vi "Check Overflows.vi"(0 "ignore overflow?":bool, 1 "clear overflow?":bool, 2 "reset":bool, 5 "overflow":bool, 7 "samples per cycle (SPC)":u32, 9 "input valid":bool, 11 "group delay (samples)":fxp<+,64,32> format="%#_42g") -> (4 "overflow?":bool)   [LabVIEW 2023]
doc: "<b>Pipeline Delay = 0</b>\n\nthis VI checks for overflows based on the input configuration. the 'overflow' is latched and must be cleared via 'clear overflow?' or 'reset'.\n\n<b>clear overflow?:</b> clear the overflow status. will immediately affect the output 'overflow?'.\n\n<b>ignore overflows:</b> indicates that overflows detected in the current cycle should be suppressed.\n\n<b>group delay (samples):</b> used to define the number of samples to ignore for unwanted DSP transients. if set to constant 0, group delay logic will not be placed."
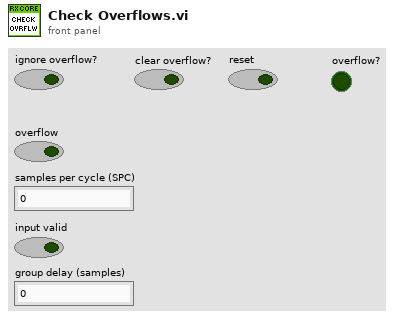
[diagram p1: front panel]
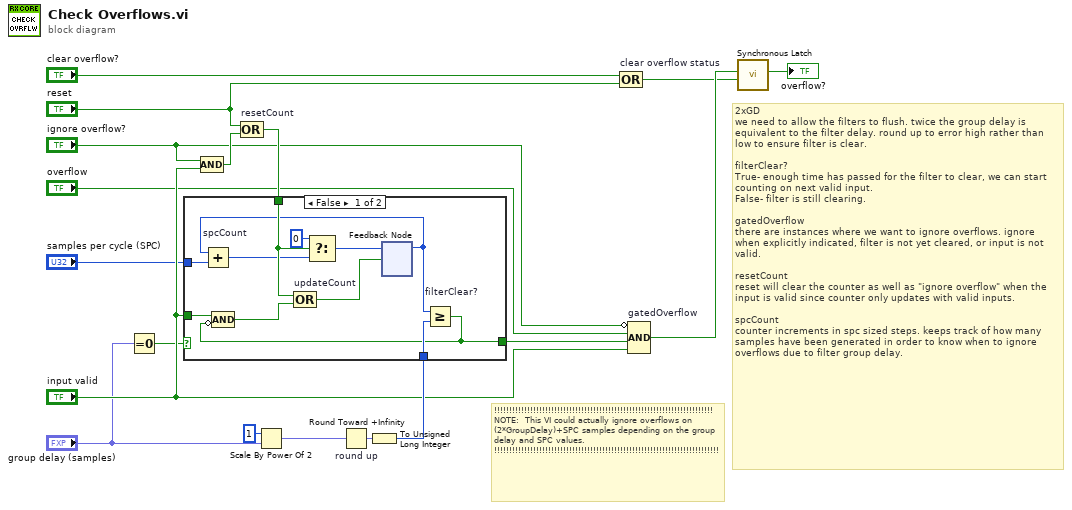
[diagram p0: block diagram]
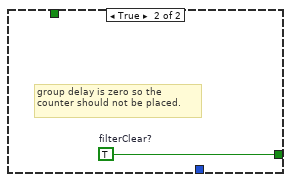
[diagram p2: hidden frame]
diagram:
  # "!!!!!!!!!!!!!!!!!!!!!!!!!!!!!!!!!!!!!!!!!!!!!!!!!!!!!!!!!!!!!!!!!!!!!!!!!\nNOTE:  This VI could actually ignore overflows on (2*GroupDelay)+SPC samples depending on the group delay and SPC values.\n!!!!!!!!!!!!!!!!!!!!!!!!!!!!!!!!!!!!!!!!!!!!!!!!!!!!!!!!!!!!!!!!!!!!!!!!!!!"
  # "2xGD\nwe need to allow the filters to flush. twice the group delay is equivalent to the filter delay. round up to error high rather than low to ensure filter is clear.\n\nfilterClear?\nTrue- enough time has passed for the filter to clear, we can start counting on next valid input.\nFalse- filter is still clearing.\n\ngatedOverflow\nthere are instances where we want to ignore overflows. ignore when explicitly indicated, filter is not yet cleared, or input is not valid.\n\nresetCount\nreset will clear the counter as well as \"ignore overflow\" when the input is valid since counter only updates with valid inputs.\n\nspcCount\ncounter increments in spc sized steps. keeps track of how many samples have been generated in order to know when to ignore overflows due to filter group delay."
  n1 = Equal To 0?(x="group delay (samples)") -> (x = 0?=w2:bool)
  n2 = Compound Arithmetic op=AND("ignore overflow?", "input valid") -> (w13:bool)
  n3 = Compound Arithmetic op=OR "resetCount"("reset", w13) -> (w12:bool)
  n4 = Scale By Power Of 2(n=i16 1, x="group delay (samples)") -> (x*2^n=w16:fxp<+,64,32>)
  n5 = Round Toward +Infinity "round up"(x=w16) -> (ceil(x): smallest int >= x=w15:fxp<+,33,33>)
  n6 = To Unsigned Long Integer(number=w15) -> (unsigned 32bit integer=w14:u32)
  n7 = case shown="False" w2 {
    tunnel: w14 -> [w29 _]
    tunnel: w12 -> [w25 _]
    tunnel: [w21 w30] -> w11
    tunnel: "input valid" -> [w20 _]
    tunnel: "samples per cycle (SPC)" -> [w19 _]
    frame False {
      n8 = feedback #1() -> (w23:u32)  [unwired: 1 in]
      n9 = Add "spcCount"(x=w23, y=w19) -> (x+y=w22:u32)
      n10 = Select(t=u32 0, s=w25, f=w22) -> (s? t:f=w27:u32)
      n11 = Greater Or Equal? "filterClear?"(x=w23, y=w29) -> (x >= y?=w21:bool)
      n12 = Compound Arithmetic op=AND(w20, invert w21) -> (w24:bool)
      n13 = Compound Arithmetic op=OR "updateCount"(w25, w24) -> (w26:bool)
      n14 = feedback-in #1(w27, w26) -> ()
    }
    frame True {
      w30 = TRUE  # filterClear?
      # "group delay is zero so the counter should not be placed."
    }
  }
  n15 = Compound Arithmetic op=OR "clear overflow status"("clear overflow?", "reset") -> (w7:bool)
  n16 = Compound Arithmetic op=AND "gatedOverflow"(invert "ignore overflow?", "overflow", w11, "input valid") -> (w8:bool)
  n17 = call <instrlib>:"Synchronous Latch.vi"("clear"=w7, "set"=w8) -> ("out"=→"overflow?":bool)  [unwired: 9 in]
